vi "Extract coordinates for nodes.vi"(2 "error in (no error)":errorcluster, 4 "Edges":T1(array[cluster]), 5 "Number of Nodes":i32) -> (0 "error out":errorcluster, 1 "Coordinates":cluster{"X":dbl, "Y":dbl}[](array[cluster]))   [LabVIEW 2009]
panel:
  out "Edges 2":T1(array[cluster])
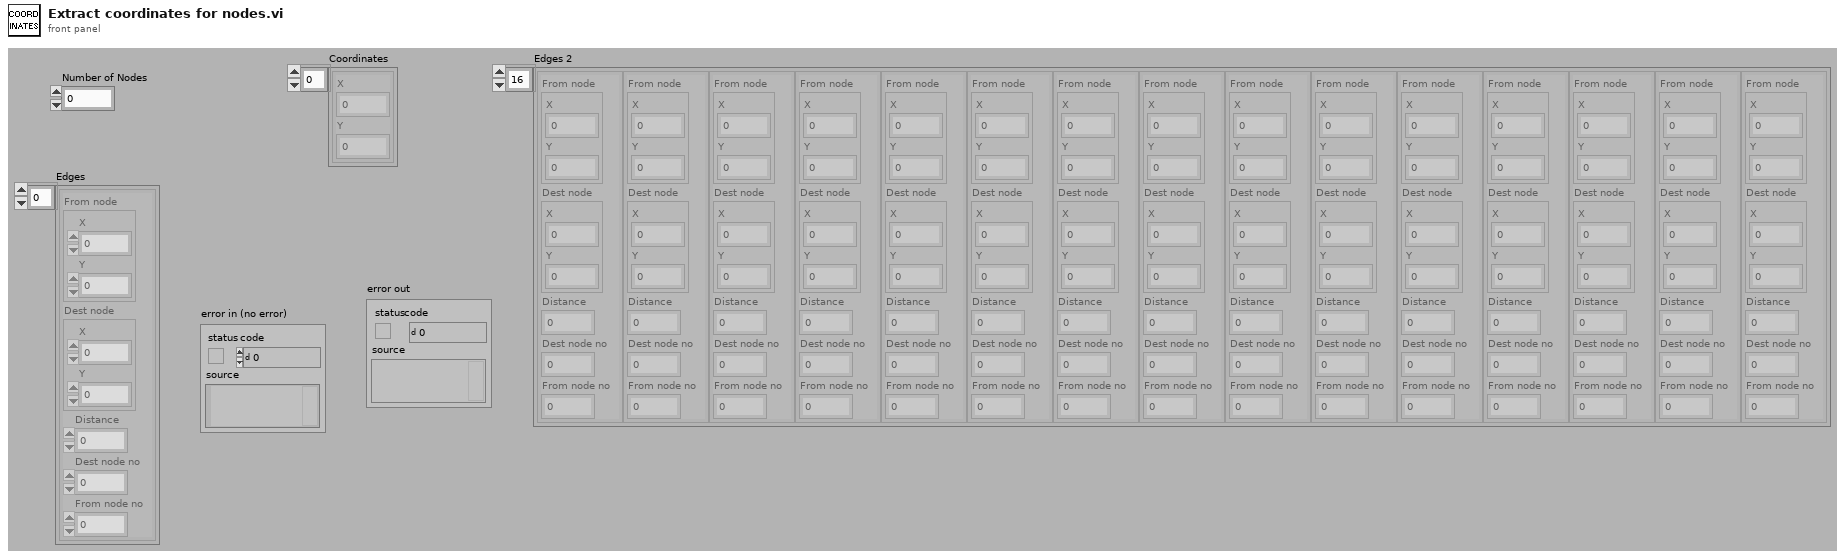
[diagram p1: front panel]
types:
  T1 = cluster{"From node":cluster{"X":dbl, "Y":dbl}, "Dest node":cluster{"X":dbl, "Y":dbl}, "Distance":dbl, "Dest node no":i32, "From node no":i32}[]
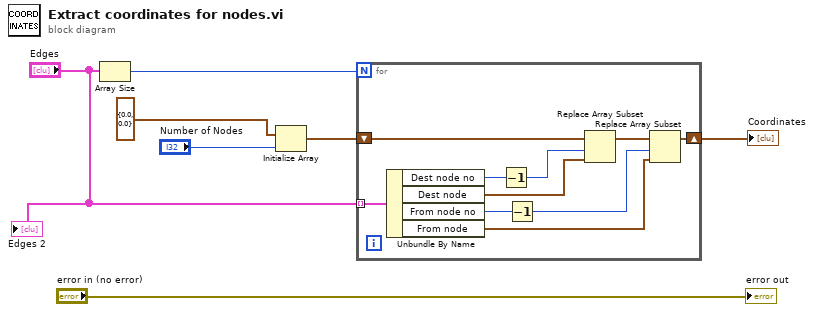
[diagram p0: block diagram]
diagram:
  n1 = Array Size(array="Edges") -> (size(s)=w7:i32)
  n2 = Initialize Array(cluster{"X":dbl, "Y":dbl} {"X"=0.0, "Y"=0.0} ("Nodes Coordinate"), "Number of Nodes") -> (w3:cluster{"X":dbl, "Y":dbl}[])
  n3 = for {
    N: w7 -> [_]
    tunnel: "Edges" -> [w17] mode=indexing
    shift-right: [w14] -> w1
    shift-left: w3 -> [w16]
    n4 = Unbundle By Name(w17) -> ("Dest node no"=w9:i32, "Dest node"=w13:cluster{"X":dbl, "Y":dbl}, "From node no"=w11:i32, "From node"=w12:cluster{"X":dbl, "Y":dbl})
    n5 = Decrement(x=w9) -> (x-1=w8:i32)
    n6 = Decrement(x=w11) -> (x-1=w10:i32)
    n7 = Replace Array Subset(array=w16, new element=w13, index=w8) -> (w15:cluster{"X":dbl, "Y":dbl}[])
    n8 = Replace Array Subset(array=w15, new element=w12, index=w10) -> (w14:cluster{"X":dbl, "Y":dbl}[])
  }
  "Coordinates" <- w1
  "error out" <- "error in (no error)"
  "Edges 2" <- "Edges"
